vi "WPI_CameraSet Frame Rate.vi"(8 "error in (no error)":errorcluster, 10 "Frame Rate (fps)":T1=30 min=1 max=30, 11 "CameraDevRef":T2) -> (0 "error out":errorcluster, 3 "CameraDevRef Out":T2)   [LabVIEW 2017]
doc: "Specifies the frequency, in frames per second, at which you want the camera you specify to capture a new set of image data.\n\nThis software is licensed. Open the labview\\readme\\WPI Robotics Library Open Source License.txt file for more information."
uses:
  <vilib>/Rock Robotics/WPI/Camera/WPI_CameraDevRef.ctl
  <vilib>/Rock Robotics/WPI/Camera/WPI_CameraFrameRate.ctl
  <vilib>/Rock Robotics/WPI/Camera/WPI_CameraSettings Operations.ctl
  <vilib>/vision/driver/NI_Vision_Acquisition_Software.lvlib
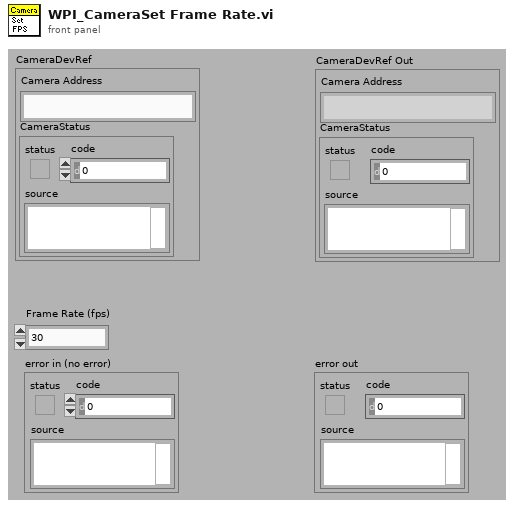
[diagram p1: front panel]
types:
  T1 = typedef "WPI_CameraFrameRate.ctl" = u32
  T2 = typedef "WPI_CameraDevRef.ctl" = cluster{"Camera Address":string, "CameraStatus":errorcluster}
  T3 = typedef "WPI_CameraSettings Operations.ctl" = enum16{"Udate FPS", "Update Compression", "Update Size", "Update White Balance", "Update Brightness", "Update Sharpness", "Update Exposure", "Update Exposure Value", "Update Color Level", "Update Exp Priority", "Update Color Enable", "Update JPG", "Update MJPG", "Read and Clear", "Read", "Init"}
  T4 = cluster{"Video Mode":u32, "Video Mode Name":string}[]
  T5 = typedef "IMAQdx.ctl" = refnum<k21>
  T6 = cluster{"Video Mode":u32, "Video Mode Name":string}
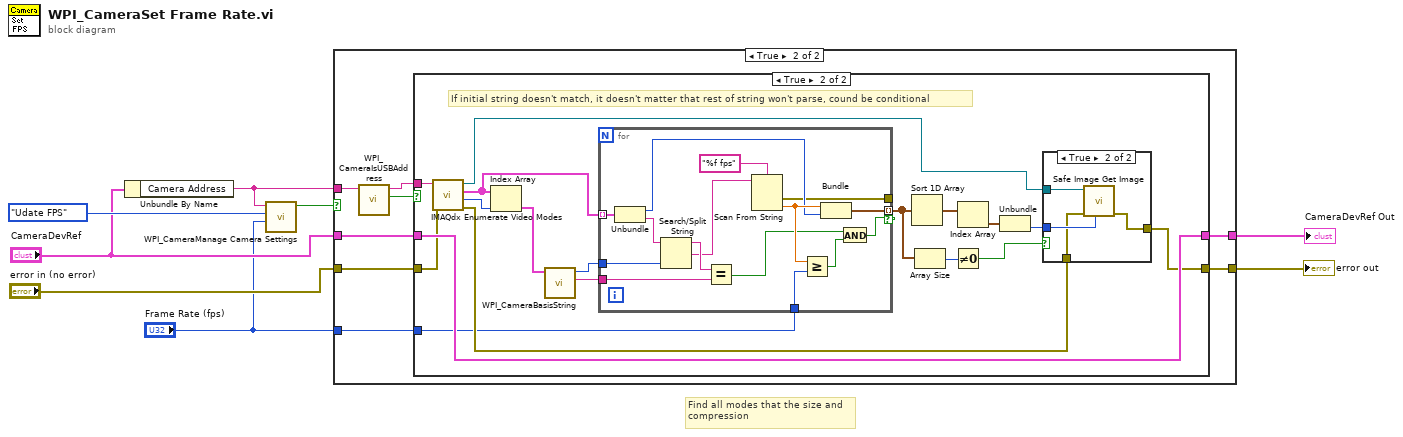
[diagram p0: block diagram]
diagram:
  # "Find all modes that the size and\ncompression"
  n1 = Unbundle By Name("CameraDevRef") -> ("Camera Address"=w7:string)
  n2 = call <vilib>:"WPI_CameraManage Camera Settings.vi"("Value"="Frame Rate (fps)", "Operation"=WPI_CameraSettings_Operations."Udate FPS", "Camera IP"=w7) -> ("Changed"=w1:bool)  [unwired: 7 in, 1 out]
  n3 = case shown="True" w1 {
    tunnel: w7 -> [_ w16]
    tunnel: [w10 w15] -> w6
    tunnel: [w9 w14] -> w5
    tunnel: "error in (no error)" -> [w9 w13]
    tunnel: "CameraDevRef" -> [w10 w12]
    tunnel: "Frame Rate (fps)" -> [_ w11]
    frame False {
    }
    frame True {
      n4 = call <vilib>:"WPI_CameraIsUSBAddress.vi"("Camera Address In"=w16) -> ("USB?"=w18:bool, "Camera Address Out"=w17:string)  [unwired: 8 in, 1 out]
      n5 = case shown="True" w18 {
        tunnel: w12 -> [w19 w36]
        tunnel: [w19 w36] -> w15
        tunnel: [w20 w35] -> w14
        tunnel: w13 -> [w20 w34]
        tunnel: w17 -> [_ w22]
        tunnel: w11 -> [_ w30]
        frame False {
        }
        frame True {
          # "If initial string doesn't match, it doesn't matter that rest of string won't parse, cound be conditional"
          n6 = call <vilib>:"IMAQdx Enumerate Video Modes.vi"("error in"=w34, "Session In"=w22) -> ("error out"=w33:errorcluster, "Current Mode"=w38:u32, "Video Modes"=w37:T4, "Session Out"=w21:T5)  [unwired: 6 in]
          n7 = Index Array(array=w37, index=w38) -> (element=w23:T6)
          n8 = call <vilib>:"WPI_CameraBasisString.vi"("Input Mode"=w23) -> ("Basis"=w32:string, "length"=w31:i32)  [unwired: 9 in]
          n9 = for {
            tunnel: w37 -> [w58] mode=indexing
            tunnel: [w45] -> w26 mode=indexing if=w46
            tunnel: w32 -> [w57]
            tunnel: w31 -> [w55]
            tunnel: w30 -> [w51]
            tunnel: [w44] -> _
            n10 = Unbundle(w58) -> ("Video Mode"=w49:u32, "Video Mode Name"=w56:string)
            n11 = Search/Split String(string=w56, offset (0)=w55) -> (substring before match=w54:string, match + rest of string=w53:string)  [unwired: 1 in, 1 out]
            n12 = Equal?(x=w54, y=w57) -> (x = y?=w47:bool)
            n13 = Scan From String(format string="%f fps", input string=w53) -> (error out=w44:errorcluster, output 1=w50:dbl)  [unwired: 3 in, 2 out]
            n14 = Greater Or Equal?(x=w50, y=w51) -> (x >= y?=w48:bool)
            n15 = Bundle(w50, "Video Mode"=w49) -> (w45:cluster{dbl, "Video Mode":u32})  [unwired: 1 in]
            n16 = And(x=w47, y=w48) -> (x .and. y?=w46:bool)
          }
          n17 = Sort 1D Array(array=w26) -> (sorted array=w29:cluster{dbl, "Video Mode":u32}[])
          n18 = Array Size(array=w26) -> (size(s)=w25:i32)
          n19 = Not Equal To 0?(x=w25) -> (x != 0?=w24:bool)
          n20 = Index Array(array=w29) -> (element=w28:cluster{dbl, "Video Mode":u32})  [unwired: 1 in]
          n21 = Unbundle(w28) -> ("Video Mode"=w27:u32)  [unwired: 1 out]
          n22 = case shown="True" w24 {
            tunnel: w27 -> [_ w42]
            tunnel: w21 -> [_ w43]
            tunnel: w33 -> [w39 w40]
            tunnel: [w39 w41] -> w35
            frame False {
            }
            frame True {
              n23 = call <vilib>:"Safe Image Get Image.vi"("Video Mode"=w42, "error in"=w40, "Session In"=w43) -> ("error out"=w41:errorcluster)  [unwired: 5 in, 3 out]
            }
          }
        }
      }
    }
  }
  "CameraDevRef Out" <- w6
  "error out" <- w5
